vi "LV Semaphore Release Destroy.vi"(8 "error in":errorcluster, 11 "semaphore":T1) -> (0 "error out":errorcluster)   [LabVIEW 2011]
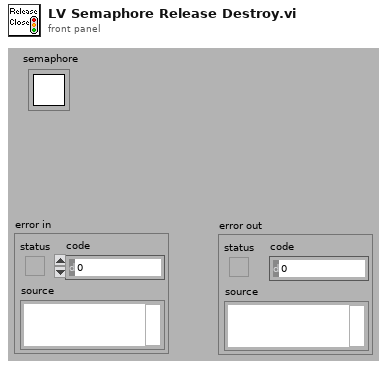
[diagram p1: front panel]
types:
  T1 = typedef "Semaphore RefNum" = refnum<k1>
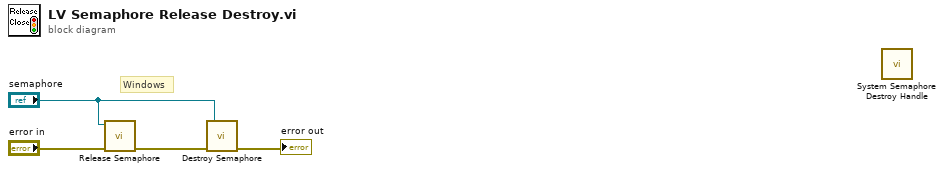
[diagram p0: block diagram]
diagram:
  # "Windows"
  n1 = call <vilib>:"Release Semaphore.vi"("error in (no error)"="error in", "semaphore"="semaphore") -> ("error out"=w1:errorcluster)  [unwired: 5 out]
  n2 = call <vilib>:"Destroy Semaphore.vi"("error in (no error)"=w1, "semaphore"="semaphore") -> ("error out"=→"error out":errorcluster)  [unwired: 5 out]
  n3 = call "System Semaphore Destroy Handle.vi"() -> ()  [unwired: 2 in, 10 out]
